vi "Get Laser State.vi"(7 "error in (no error)":errorcluster, 10 "object in":refnum<class "Laser Ethernet Rack.lvclass">) -> (0 "error out":errorcluster, 3 "object out":refnum<class "Laser Ethernet Rack.lvclass">)   [LabVIEW 2023, in "Laser Ethernet Rack.lvclass"]
uses:
  Laser Ethernet Rack.lvclass
  Laser Ethernet Rack.lvclass/Laser Ethernet Rack.ctl
  Laser_Ethernet_class/Laser_Ethernet.lvclass
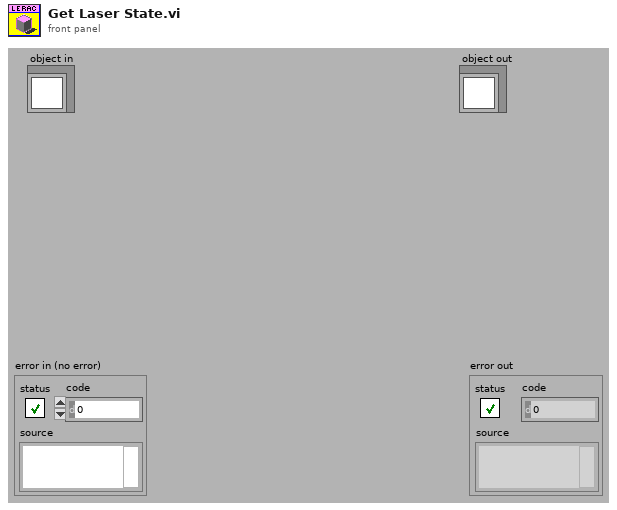
[diagram p1: front panel]
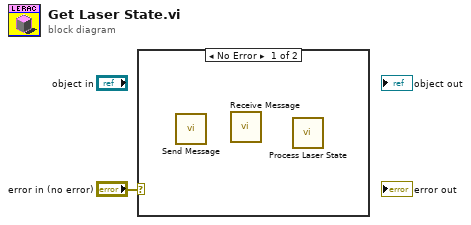
[diagram p0: block diagram]
diagram:
  n1 = case shown="No Error" "error in (no error)" {
    frame No Error {
      n2 = call "Send Message.vi"() -> ()  [unwired: 10 in, 2 out]
      n3 = call "Receive Message.vi"() -> ()  [unwired: 9 in, 3 out]
      n4 = call-dynamic "Process Laser State.vi"() -> ()  [unwired: 9 in, 2 out]
    }
    frame Error {
    }
  }
